vi "LSMcontroller_v58.vi"() -> ()   [LabVIEW 2015] (continued)
                                n1730 = Divide(x=1.0 ("Digital DC (%)"), y=w4415) -> (x/y=w4417:dbl)
                                n1731 = Multiply(x=100.0, y=w4417) -> (x*y=w4414:dbl)
                                n1732 = Bundle By Name(cluster=w4431, "Digital DC (%)"=w4414, "Digital phase"=w4426, "Digital Freq (Hz)"=w4422, "Sampling frequency (Hz)"=w4419, "Digital time offset (s)"=w4426, "padding value"=0.0, "matlab wave file"=path "LT", "DOtab"=0.0) -> (w4429:T20)
                                n1733 = Build Array(w4429) -> (w4428:T19)
                                n1734 = call "waveformparamsv2.vi"("command"="add DO", "add DO"=w4428) -> ()  [unwired: 3 in, 3 out]
                                }
                                frame 2 {
                                n1735 = call "waveformparamsv2.vi"("command"="get") -> ("Params out"=w4441:T16)  [unwired: 4 in, 2 out]
                                n1736 = in-place {
                                in-place-border: w4439 -> [w4445]
                                in-place-border: [w4444] -> w4438
                                n1737 = in-place-cluster #30(w4441) -> ("DO parameters"=w4447:T19)
                                n1738 = Delete From Array(array=w4447, length=1, index=w4445) -> (deleted portion=w4444:T19, array with subset deleted=w4446:T19)
                                n1739 = in-place-cluster #30("DO parameters"=w4446) -> (w4440:T16)
                                }
                                n1740 = call "waveformparamsv2.vi"("command"="set", "Params in"=w4440) -> ()  [unwired: 3 in, 3 out]
                                }
                                frame 3, Default {
                                }
                                frame 0 {
                                n1741 = local read "Measurement"() -> (w4453:T5)
                                n1742 = To Unsigned Long Integer(number=w4453) -> (unsigned 32bit integer=w4452:u32)
                                n1743 = case shown="5..7" w4452 {
                                tunnel: w4451 -> [_ w4455]
                                tunnel: [_ w4454] -> w4450
                                frame 0..4, Default {
                                }
                                frame 5..7 {
                                n1744 = stacked-sequence {
                                tunnel: w4455 -> [w4457 w4466]
                                tunnel: [w4456 _] -> w4454
                                frame #0 {
                                n1745 = call "waveformparamsv2.vi"("command"="get") -> ("Params out"=w4459:T16)  [unwired: 4 in, 2 out]
                                n1746 = Unbundle By Name(w4459) -> ("DO parameters"=w4460:T19)
                                n1747 = Index Array(array=w4460, index=w4457) -> (element=w4456:T20)
                                }
                                frame #1 {
                                w4474 = 0.0 ("padding value")
                                n1748 = call "2pparameters.vi"("command"="get") -> ("params out"=w4472:T12)  [unwired: 1 in]
                                n1749 = Unbundle By Name(w4472) -> ("srate"=w4470:sgl, "Pel"=w4471:sgl)
                                n1750 = To Double Precision Float(number=w4470) -> (double precision float=w4468:dbl)
                                n1751 = To Double Precision Float(number=w4470) -> (double precision float=w4469:dbl)
                                n1752 = To Double Precision Float(number=w4471) -> (double precision float=w4464:dbl)
                                n1753 = Divide(x=1.0 ("Digital DC (%)"), y=w4464) -> (x/y=w4463:dbl)
                                n1754 = Multiply(x=100.0, y=w4463) -> (x*y=w4462:dbl)
                                n1755 = Divide(x=w4469, y=w4464) -> (x/y=w4467:dbl)
                                n1756 = call "replace DO wf param.vi"("Digital Freq (Hz)"=w4467, "Digital DC (%)"=w4462, "Digital phase"=w4474, "Sampling frequency (Hz)"=w4468, "Digital time offset (s)"=w4474, "index of DO wave"=w4466, "padding value"=w4474, "matlab wave file"=path "LT" ("matlab wave number")) -> ()  [unwired: 3 in]
                                }
                                }
                                }
                                }
                                n1757 = Build Array(w4450) -> (w4449:T19)
                                }
                                }
                                }
                                frame #9 {
                                n1758 = Build Array(w4479, w4478) -> (w4481:bool[])
                                n1759 = Boolean Array To Number(Boolean array=w4481) -> (number=w4480:u32)
                                n1760 = case shown="0" w4480 {
                                tunnel: w4477 -> [_ w4533 _ w4537]
                                tunnel: [_ w4528 _ w4534] -> w4476
                                frame 1 {
                                n1761 = call "2pparameters.vi"("command"="get") -> ("params out"=w4488:T12)  [unwired: 1 in]
                                n1762 = Unbundle By Name(w4488) -> ("wavdet"=w4489:bool, "Pel"=w4491:sgl, "refwfsize"=w4492:dbl, "Pel"=w4490:sgl)
                                n1763 = call "waveformsDObuffer.vi"("command"="get") -> ("DO wf out"=w4484:digitalwaveform[])  [unwired: 1 in]
                                n1764 = case shown="True" w4489 {
                                tunnel: [w4496 w4509] -> w4486
                                tunnel: w4490 -> [w4505 w4524]
                                tunnel: w4491 -> [w4495 w4515]
                                tunnel: w4492 -> [_ w4521]
                                frame False {
                                w4499 = u16 0 items=["unsigned binary", "offset binary", "2's complement"] ("data format (offset binary)")
                                n1765 = Initialize Array(sgl 0.0, w4495) -> (w4502:sgl[])
                                n1766 = Replace Array Subset(array=w4502, new element=sgl 1.0, index=0) -> (w4500:sgl[])
                                n1767 = Reciprocal(x=w4505) -> (1/x=w4506:sgl)
                                n1768 = Bundle By Name("Y"=w4500, "dt"=w4506) -> (w4497:waveform(sgl))  [unwired: 1 in]
                                n1769 = call-poly <vilib>:"Analog to Digital.vi"("data format (offset binary)"=w4499, "compress digital (T)"=TRUE, "full-scale range (pk-pk)"=1.0, "resolution (16 bit)"=1, "analog waveform"=w4497) -> ("digital waveform"=w4496:digitalwaveform)  [unwired: 3 in, 3 out]
                                }
                                frame True {
                                w4512 = u16 0 items=["unsigned binary", "offset binary", "2's complement"] ("data format (offset binary)")
                                n1770 = To Double Precision Float(number=w4515) -> (double precision float=w4522:dbl)
                                n1771 = Initialize Array(sgl 0.0, w4515) -> (w4517:sgl[])
                                n1772 = Divide(x=w4521, y=w4522) -> (x/y=w4519:dbl)
                                n1773 = Round Toward +Infinity(x=w4519) -> (ceil(x): smallest int >= x=w4520:dbl)
                                n1774 = Replace Array Subset(array=w4517, new element=sgl 1.0, index=0) -> (w4514:sgl[])
                                n1775 = for {
                                N: w4520 -> [_]
                                tunnel: w4514 -> [w4526]
                                tunnel: [w4526] -> w4523 mode=concatenating
                                }
                                n1776 = Reciprocal(x=w4524) -> (1/x=w4525:sgl)
                                n1777 = Bundle By Name("Y"=w4523, "dt"=w4525) -> (w4510:waveform(sgl))  [unwired: 1 in]
                                n1778 = call-poly <vilib>:"Analog to Digital.vi"("data format (offset binary)"=w4512, "compress digital (T)"=TRUE, "full-scale range (pk-pk)"=1.0, "resolution (16 bit)"=1, "analog waveform"=w4510) -> ("digital waveform"=w4509:digitalwaveform)  [unwired: 3 in, 3 out]
                                }
                                }
                                n1779 = Build Array (concatenate)(w4484, w4486) -> (w4482:digitalwaveform[])
                                n1780 = call "waveformsDObuffer.vi"("DO wf in"=w4482, "command"="set") -> ()  [unwired: 1 out]
                                }
                                frame 2 {
                                n1781 = call "waveformsDObuffer.vi"("command"="get") -> ("DO wf out"=w4530:digitalwaveform[])  [unwired: 1 in]
                                n1782 = Delete From Array(array=w4530, length=1, index=w4533) -> (deleted portion=w4528:digitalwaveform[], array with subset deleted=w4527:digitalwaveform[])
                                n1783 = call "waveformsDObuffer.vi"("DO wf in"=w4527, "command"="set") -> ()  [unwired: 1 out]
                                }
                                frame 3, Default {
                                }
                                frame 0 {
                                n1784 = local read "Measurement"() -> (w4536:T5)
                                n1785 = To Unsigned Long Integer(number=w4536) -> (unsigned 32bit integer=w4535:u32)
                                n1786 = case shown="5..7" w4535 {
                                tunnel: w4537 -> [_ w4540]
                                tunnel: [_ w4539] -> w4534
                                frame 0..4, Default {
                                }
                                frame 5..7 {
                                n1787 = call "2pparameters.vi"("command"="get") -> ("params out"=w4547:T12)  [unwired: 1 in]
                                n1788 = Unbundle By Name(w4547) -> ("wavdet"=w4548:bool, "Pel"=w4550:sgl, "refwfsize"=w4551:dbl, "srateAODO"=w4549:sgl)
                                n1789 = call "waveformsDObuffer.vi"("command"="get") -> ("DO wf out"=w4541:digitalwaveform[])  [unwired: 1 in]
                                n1790 = Index Array(array=w4541, index=w4540) -> (element=w4542:digitalwaveform)
                                n1791 = case shown="True" w4548 {
                                tunnel: [w4555 w4568] -> w4545
                                tunnel: w4549 -> [w4564 w4583]
                                tunnel: w4550 -> [w4554 w4574]
                                tunnel: w4551 -> [_ w4580]
                                frame False {
                                w4558 = u16 0 items=["unsigned binary", "offset binary", "2's complement"] ("data format (offset binary)")
                                n1792 = Initialize Array(sgl 0.0, w4554) -> (w4561:sgl[])
                                n1793 = Replace Array Subset(array=w4561, new element=sgl 1.0, index=0) -> (w4559:sgl[])
                                n1794 = Reciprocal(x=w4564) -> (1/x=w4565:sgl)
                                n1795 = Bundle By Name("Y"=w4559, "dt"=w4565) -> (w4556:waveform(sgl))  [unwired: 1 in]
                                n1796 = call-poly <vilib>:"Analog to Digital.vi"("data format (offset binary)"=w4558, "compress digital (T)"=TRUE, "full-scale range (pk-pk)"=1.0, "resolution (16 bit)"=1, "analog waveform"=w4556) -> ("digital waveform"=w4555:digitalwaveform)  [unwired: 3 in, 3 out]
                                }
                                frame True {
                                w4571 = u16 0 items=["unsigned binary", "offset binary", "2's complement"] ("data format (offset binary)")
                                n1797 = To Double Precision Float(number=w4574) -> (double precision float=w4581:dbl)
                                n1798 = Initialize Array(sgl 0.0, w4574) -> (w4576:sgl[])
                                n1799 = Divide(x=w4580, y=w4581) -> (x/y=w4578:dbl)
                                n1800 = Round Toward +Infinity(x=w4578) -> (ceil(x): smallest int >= x=w4579:dbl)
                                n1801 = Replace Array Subset(array=w4576, new element=sgl 1.0, index=0) -> (w4573:sgl[])
                                n1802 = for {
                                N: w4579 -> [_]
                                tunnel: w4573 -> [w4585]
                                tunnel: [w4585] -> w4582 mode=concatenating
                                }
                                n1803 = Reciprocal(x=w4583) -> (1/x=w4584:sgl)
                                n1804 = Bundle By Name("Y"=w4582, "dt"=w4584) -> (w4569:waveform(sgl))  [unwired: 1 in]
                                n1805 = call-poly <vilib>:"Analog to Digital.vi"("data format (offset binary)"=w4571, "compress digital (T)"=TRUE, "full-scale range (pk-pk)"=1.0, "resolution (16 bit)"=1, "analog waveform"=w4569) -> ("digital waveform"=w4568:digitalwaveform)  [unwired: 3 in, 3 out]
                                }
                                }
                                n1806 = Build Array(w4542) -> (w4539:digitalwaveform[])
                                n1807 = Replace Array Subset(array=w4541, new element=w4545, index=w4540) -> (w4538:digitalwaveform[])
                                n1808 = call "waveformsDObuffer.vi"("DO wf in"=w4538, "command"="set") -> ()  [unwired: 1 out]
                                }
                                }
                                }
                                }
                                }
                                frame #10 {
                                n1809 = local read "Meastab"() -> (w4599:enum32{"X-Y Image", "Linescan", "Timetrace"})
                                n1810 = property on="refwf" class="Ring (strict)"() -> ("RingText.Text"=w4596:string)  [unwired: 2 in, 2 out]
                                n1811 = case shown="\"Timetrace\"" w4599 {
                                tunnel: [w4601 w4602] -> w4600
                                frame "X-Y Image", Default {
                                n1812 = local read "Sampling rate"() -> (w4601:dbl)
                                }
                                frame "Timetrace" {
                                n1813 = local read "srateAODOtt"() -> (w4602:dbl)
                                }
                                }
                                n1814 = call "waveformsAObuffer.vi"("command"="get") -> ("AO wf out"=w4589:waveform(dbl)[])  [unwired: 1 in]
                                n1815 = local read "wavdet"() -> (w4597:bool)
                                n1816 = call "waveformsDObuffer.vi"("command"="get") -> ("DO wf out"=w4593:digitalwaveform[])  [unwired: 1 in]
                                n1817 = call "correctwaveformsizetemp.vi"("new sampling frequency (Hz)"=w4600, "start"=TRUE, "reference waveforms to"=w4596, "Analog waveforms in"=w4589, "stop"=FALSE, "Digital waveforms in"=w4593) -> ("analog wf out"=w4595:waveform(dbl)[], "Digital wf out"=w4588:digitalwaveform[], "measpoints"=w4598:i32)
                                n1818 = call "waveformsDObuffer.vi"("DO wf in"=w4588, "command"="set") -> ()  [unwired: 1 out]
                                n1819 = call "waveformsAObuffer.vi"("AO wf in"=w4595, "command"="set") -> ()  [unwired: 1 out]
                                n1820 = case shown="True" w4597 {
                                tunnel: w4598 -> [_ w4605]
                                tunnel: w4588 -> [_ w4603]
                                frame False {
                                }
                                frame True {
                                n1821 = local write "# of frames"(w4605) -> ()
                                n1822 = call "GetNumCamFramesv2.vi"("Digital Waveform Graph"=w4603) -> ("Numeric"=w4604:i32)  [unwired: 10 in]
                                n1823 = local write "Total Camera Frames"(w4604) -> ()
                                }
                                }
                                }
                                }
                              }
                              frame #7 {
                                # "Disabled for conversion to 64 bit"
                                n1824 = disable-structure shown="Disabled" {
                                frame Disabled {
                                n1825 = local read "Measurement"() -> (w4607:T5)
                                n1826 = case shown="\"Lifetime (scan)\"" w4607 {
                                frame "X-Y-t movie", Default {
                                }
                                frame "Lifetime (scan)" {
                                # "total acquisition time"
                                n1827 = call "2pparameters.vi"("command"="get") -> ("params out"=w4615:T12)  [unwired: 1 in]
                                n1828 = Unbundle By Name(w4615) -> ("measpoints"=w4609:i32, "srateAODO"=w4630:sgl)
                                n1829 = Divide(x=w4609, y=w4630) -> (x/y=w4608:sgl)
                                n1830 = local read "min phot"() -> (w4625:u32)
                                n1831 = local read "expected c/s"() -> (w4626:dbl)
                                n1832 = Multiply(x=w4608, y=1000.0) -> (x*y=w4618:dbl)
                                n1833 = local read "Ch1 ZeroX"() -> (w4623:i32)
                                n1834 = local read "truncate"() -> (w4624:u32)
                                n1835 = To Long Integer(number=w4618) -> (32bit integer=w4627:i32)
                                n1836 = To Long Integer(number=w4626) -> (32bit integer=w4628:i32)
                                n1837 = local read "Number of Bins"() -> (w4619:u32)
                                n1838 = local read "Ch1 Level"() -> (w4621:i32)
                                n1839 = local read "Ch0 ZeroX"() -> (w4622:i32)
                                n1840 = local write "Acquisition time"(w4627) -> ()
                                n1841 = local read "Ch0 Level"() -> (w4620:i32)
                                n1842 = call "lifetimeparameters.vi"("command"="get") -> ("Params out"=w4613:T21)  [unwired: 1 in]
                                n1843 = Add(x=100, y=w4627) -> (x+y=w4617:i32)
                                n1844 = Bundle By Name(cluster=w4613, "acq time"=w4617, "acq rate"=w4628, "# bins"=w4619, "Ch0 Level"=w4620, "Ch1 Level"=w4621, "Ch0 ZeroX"=w4622, "Ch1 ZeroX"=w4623, "min photons"=w4625, "truncate"=w4624) -> (w4612:T21)
                                n1845 = local write "Acquisition rate"(w4628) -> ()
                                n1846 = call "lifetimeparameters.vi"("Params in"=w4612, "command"="set") -> ()  [unwired: 1 out]
                                }
                                }
                                }
                                frame Enabled {
                                }
                                }
                                n1847 = local write "64bit disabled"(TRUE ("64bit disabled")) -> ()
                              }
                              frame #8 {
                                n1848 = call "2pparameters.vi"("command"="get") -> ("params out"=w4641:T12)  [unwired: 1 in]
                                n1849 = Unbundle By Name(w4641) -> ("refreshbuffer"=w4639:i32, "srate"=w4640:sgl)
                                n1850 = local read "wavdet"() -> (w4631:bool)
                                n1851 = To Double Precision Float(number=w4640) -> (double precision float=w4643:dbl)
                                n1852 = To Double Precision Float(number=w4639) -> (double precision float=w4634:dbl)
                                n1853 = case shown="False" w4631 {
                                tunnel: [w4648 w4649] -> w4633
                                frame False {
                                w4648 = 10123 items=["Finite Samples"=10178, "Continuous Samples"=10123, "Hardware Timed Single Point"=12522] ("sample mode")
                                }
                                frame True {
                                w4649 = 10123 items=["Finite Samples"=10178, "Continuous Samples"=10123, "Hardware Timed Single Point"=12522] ("sample mode")
                                }
                                }
                                n1854 = Divide(x=w4634, y=w4643) -> (x/y=w4647:dbl)
                                n1855 = Multiply(x=w4647, y=2.0) -> (x*y=w4644:dbl)
                                n1856 = Max & Min(x=w4644, y=10.0) -> (max(x,y)=w4635:dbl)  [unwired: 1 out]
                                n1857 = call "2pparameters.vi"("command"="get") -> ("params out"=w4638:T12)  [unwired: 1 in]
                                n1858 = Bundle By Name(cluster=w4638, "timeout"=w4635, "sample mode"=w4633) -> (w4636:T12)
                                n1859 = call "2pparameters.vi"("Params in"=w4636, "command"="set") -> ()  [unwired: 1 out]
                              }
                            }
                          }
                          frame #1 {
                            # "Disabled for conversion to 64 bit"
                            n1860 = call "prepAO_img.vi"() -> ("Terminal Name with Device Prefix"=w4651:tag)
                            n1861 = call "prepDO_img.vi"() -> ()  [unwired: 2 in]
                            n1862 = call "prepAI_img.vi"("triggersource"=w4651) -> ()  [unwired: 2 in]
                            n1863 = call "prepCI_img.vi"("ArmStart.DigEdge.Src"=w4651) -> ()  [unwired: 1 in]
                            n1864 = disable-structure shown="Disabled" {
                              frame Disabled {
                                n1865 = local read "Measurement"() -> (w4652:T5)
                                n1866 = case shown="\"Lifetime (contour)\"" w4652 {
                                frame "X-Y-t movie", Default {
                                }
                                frame "Lifetime (contour)" {
                                n1867 = stacked-sequence {
                                frame #0 {
                                n1868 = call "PH-temp.vi"("String"="clear" ("command")) -> ()  [unwired: 2 in, 2 out]
                                n1869 = call "PH-temp-raw.vi"("command"="empty") -> ()  [unwired: 1 in, 1 out]
                                }
                                frame #1 {
                                n1870 = call "calib.vi"() -> ()  [unwired: 1 in]
                                }
                                frame #2 {
                                n1871 = call "setup.vi"() -> ()  [unwired: 1 in]
                                }
                                }
                                }
                                }
                              }
                              frame Enabled {
                              }
                            }
                            n1872 = local write "64bit disabled"(TRUE ("64bit disabled")) -> ()
                          }
                          frame #2 {
                            n1873 = local read "save\ndata"() -> (w4655:bool)
                            n1874 = case shown="True" w4655 {
                              tunnel: w4656 -> [_ w4660]
                              frame False {
                              }
                              frame True {
                                n1875 = local read "filename prefix"() -> (w4658:string)
                                n1876 = local read "data dir"() -> (w4659:path)
                                n1877 = call "preparebinaryfiles.vi"("filename prefix"=w4658, "data dir"=w4659, "timestamp"=w4660) -> ("full-filename"=w4657:string)  [unwired: 1 in]
                                n1878 = local write "full-filename"(w4657) -> ()
                              }
                            }
                            n1879 = call "preptempbuffers_tt.vi"() -> ()  [unwired: 12 in]
                          }
                          frame #3 {
                            n1880 = local read "wavdet"() -> (w4661:bool)
                            n1881 = case shown="False" w4661 {
                              frame False {
                                n1882 = disable-structure shown="Disabled" {
                                frame Disabled {
                                n1883 = call "2pparameters.vi"("command"="get") -> ("params out"=w4663:T12)  [unwired: 1 in]
                                n1884 = Unbundle By Name(w4663) -> ("autoshutter"=w4664:bool)
                                n1885 = case shown="True" w4664 {
                                frame False {
                                }
                                frame True {
                                n1886 = call "shuttercontrol.vi"("command"="open") -> ()  [unwired: 1 in, 1 out]
                                }
                                }
                                }
                                frame Enabled {
                                }
                                }
                              }
                              frame True {
                              }
                            }
                          }
                          frame #4 {
                            n1887 = flat-sequence {
                              frame #0 {
                                # "Disabled for conversion to 64 bit"
                                n1888 = disable-structure shown="Disabled" {
                                frame Disabled {
                                n1889 = local read "Measurement"() -> (w4667:T5)
                                n1890 = case shown="\"Lifetime (contour)\"" w4667 {
                                frame "X-Y-t movie", Default {
                                }
                                frame "Lifetime (contour)" {
                                n1891 = call "runLT_img.vi"() -> ()  [unwired: 1 in]
                                }
                                }
                                }
                                frame Enabled {
                                }
                                }
                                n1892 = local write "64bit disabled"(TRUE ("64bit disabled")) -> ()
                              }
                              frame #1 {
                                n1893 = call "runAI_img.vi"() -> ()  [unwired: 12 in]
                                n1894 = call "runCI.vi"() -> ()  [unwired: 12 in]
                                n1895 = call "runDO_img.vi"() -> ()  [unwired: 12 in]
                              }
                              frame #2 {
                                n1896 = call "runAO_img.vi"() -> ()  [unwired: 12 in]
                              }
                            }
                          }
                          frame #5 {
                            # "Disabled for conversion to 64 bit"
                            n1897 = disable-structure shown="Disabled" {
                              disable-tunnel: w4669 -> [w4670 _]
                              frame Disabled {
                                w4673 = u16 0 items=["Stream to disk", "Post process", "real time process"] ("Ring")
                                n1898 = local read "T3R Data processing"() -> (w4672:u16)
                                n1899 = Equal?(x=w4672, y=w4673) -> (x = y?=w4671:bool)
                                n1900 = local read "save\ndata"() -> (w4675:bool)
                                n1901 = local read "Measurement"() -> (w4676:T5)
                                n1902 = And(x=w4675, y=w4671) -> (x .and. y?=w4674:bool)
                                n1903 = case shown="\"Lifetime (contour)\"" w4676 {
                                tunnel: w4670 -> [_ w4680]
                                tunnel: w4674 -> [_ w4678]
                                frame "X-Y-t movie", Default {
                                }
                                frame "Lifetime (contour)" {
                                n1904 = case shown="True" w4678 {
                                selector: w4678 -> [w4681 w4686]
                                tunnel: w4680 -> [_ w4684]
                                tunnel: [path "" ("appended path") w4687] -> w4679
                                tunnel: [w4681 w4686] -> w4677
                                frame False {
                                }
                                frame True {
                                n1905 = local read "filename prefix"() -> (w4685:string)
                                n1906 = local read "data dir"() -> (w4688:path)
                                n1907 = call "generatedatafilename.vi"("timestamp"=w4684, "filename prefix in"=w4685) -> ("full-filename"=w4683:string)
                                n1908 = Concatenate Strings(w4683, ".lvpt3contour" ("string")) -> (w4690:string)
                                n1909 = Build Path(base path=w4688, name or relative path=w4690) -> (appended path=w4687:path)
                                }
                                }
                                n1910 = call "collectLT_res_v1.vi"("stream?"=w4677, "data file"=w4679) -> ()  [unwired: 2 out]
                                }
                                }
                              }
                              frame Enabled {
                              }
                            }
                            n1911 = while {
                              i -> [w4693]
                              stop <- w4691 stop-if-true
                              n1912 = local read "Stop"() -> (w4701:bool)
                              n1913 = local read "Exit"() -> (w4700:bool)
                              n1914 = Increment(x=w4693) -> (x+1=w4692:i32)
                              n1915 = local write "points recorded"(w4692) -> ()
                              n1916 = Or(x=w4701, y=w4700) -> (x .or. y?=w4699:bool)
                              n1917 = case shown="False" w4699 {
                                frame False {
                                n1918 = stacked-sequence {
                                frame #0 {
                                n1919 = call "collectAI_tt_V2.vi"() -> ()  [unwired: 4 in]
                                n1920 = call "collectCI_tt.vi"() -> ("size(s)"=w4708:i32)  [unwired: 3 in]
                                n1921 = local write "scol"(w4708) -> ()
                                }
                                frame #1 {
                                n1922 = local read "Live"() -> (w4709:bool)
                                n1923 = case shown="True" w4709 {
                                frame False {
                                }
                                frame True {
                                n1924 = local read "graph1list"() -> (w4716:u16)
                                n1925 = local read "graph2list"() -> (w4715:u16)
                                n1926 = To Unsigned Word Integer(number=w4716) -> (unsigned 16bit integer=w4714:u16)
                                n1927 = To Unsigned Word Integer(number=w4715) -> (unsigned 16bit integer=w4713:u16)
                                n1928 = call "dattotrace.vi"("graph2list"=w4713, "Current Average"=sgl 1.0, "graph1list"=w4714) -> ("trace2array out"=w4711:sgl[], "trace1array out"=w4722:sgl[])
                                n1929 = local read "bin"() -> (w4723:dbl)
                                n1930 = script code="data=reshape(datain,[bin length(datain)./bin]);\ndataout=mean(data,1);\ndata2=reshape(datain2,[bin length(datain2)./bin]);\ndataout2=mean(data2,1);"("bin"=w4723, "datain"=w4722, "datain2"=w4711) -> ("dataout"=w4721:dbl[], "dataout2"=w4710:dbl[])  [unwired: 1 in, 1 out]
                                n1931 = Array Size(array=w4710) -> (size(s)=w4724:i32)
                                n1932 = Divide(x=w4724, y=2) -> (x/y=w4726:dbl)
                                n1933 = Round To Nearest(number=w4726) -> (nearest integer value=w4728:dbl)
                                n1934 = Array Size(array=w4721) -> (size(s)=w4733:i32)
                                n1935 = Delete From Array(array=w4710, length=w4728, index=0) -> (deleted portion=w4719:dbl[], array with subset deleted=w4720:dbl[])
                                n1936 = Divide(x=w4733, y=2) -> (x/y=w4731:dbl)
                                n1937 = Round To Nearest(number=w4731) -> (nearest integer value=w4729:dbl)
                                n1938 = Delete From Array(array=w4721, length=w4729, index=0) -> (deleted portion=w4718:dbl[], array with subset deleted=w4717:dbl[])
                                n1939 = local write "graph2"(w4717) -> ()
                                n1940 = local write "graph1"(w4718) -> ()
                                n1941 = local write "graph3"(w4719) -> ()
                                n1942 = local write "graph4"(w4720) -> ()
                                }
                                }
                                }
                                frame #2 {
                                n1943 = local read "save\ndata"() -> (w4734:bool)
                                n1944 = case shown="True" w4734 {
                                frame False {
                                }
                                frame True {
                                n1945 = call "savebinaryfiles.vi"() -> ()  [unwired: 1 in]
                                }
                                }
                                }
                                }
                                }
                                frame True {
                                }
                              }
                              n1946 = local read "continuous"() -> (w4696:bool)
                              n1947 = case shown="False" w4696 {
                                tunnel: w4692 -> [w4706 _]
                                tunnel: [w4705 FALSE] -> w4694
                                frame False {
                                n1948 = call "2pparameters.vi"("command"="get") -> ("params out"=w4703:T12)  [unwired: 1 in]
                                n1949 = Unbundle By Name(w4703) -> ("tt_cycles"=w4702:i32)
                                n1950 = Greater Or Equal?(x=w4706, y=w4702) -> (x >= y?=w4705:bool)
                                }
                                frame True {
                                }
                              }
                              n1951 = local read "Stop"() -> (w4698:bool)
                              n1952 = local read "Exit"() -> (w4697:bool)
                              n1953 = Or(x=w4698, y=w4697) -> (x .or. y?=w4695:bool)
                              n1954 = Or(x=w4695, y=w4694) -> (x .or. y?=w4691:bool)
                            }
                            n1955 = local write "64bit disabled"(TRUE ("64bit disabled")) -> ()
                          }
                          frame #6 {
                            # "Disabled for conversion to 64 bit"
                            n1956 = local read "Measurement"() -> (w4737:T5)
                            n1957 = disable-structure shown="Disabled" {
                              disable-tunnel: w4737 -> [w4739 _]
                              disable-tunnel: w4736 -> [w4738 _]
                              frame Disabled {
                                n1958 = case shown="\"Lifetime (contour)\"" w4739 {
                                tunnel: w4738 -> [_ w4740]
                                frame "X-Y-t movie", Default {
                                }
                                frame "Lifetime (contour)" {
                                n1959 = stacked-sequence {
                                tunnel: w4740 -> [_ w4741]
                                frame #0 {
                                n1960 = flat-sequence {
                                frame #0 {
                                n1961 = call "stoperaseLT_img.vi"() -> ()  [unwired: 1 in]
                                }
                                }
                                }
                                frame #1 {
                                w4744 = u16 0 items=["Stream to disk", "Post process", "real time process"] ("Ring")
                                n1962 = local read "T3R Data processing"() -> (w4743:u16)
                                n1963 = local read "save\ndata"() -> (w4746:bool)
                                n1964 = Equal?(x=w4743, y=w4744) -> (x = y?=w4742:bool)
                                n1965 = Not(x=w4742) -> (.not. x?=w4747:bool)
                                n1966 = And(x=w4746, y=w4747) -> (x .and. y?=w4745:bool)
                                n1967 = case shown="True" w4745 {
                                tunnel: w4741 -> [_ w4748]
                                frame False {
                                }
                                frame True {
                                n1968 = local read "filename prefix"() -> (w4749:string)
                                n1969 = local read "data dir"() -> (w4765:path)
                                n1970 = call "2pparameters.vi"("command"="get") -> ("params out"=w4760:T12)  [unwired: 1 in]
                                n1971 = call "generatedatafilename.vi"("timestamp"=w4748, "filename prefix in"=w4749) -> ("full-filename"=w4750:string)
                                n1972 = Unbundle By Name(w4760) -> ("srate"=w4758:sgl, "Pel"=w4757:sgl, "measpoints"=w4755:i32)
                                n1973 = Concatenate Strings(w4750, ".lvpt3contour" ("string")) -> (w4763:string)
                                n1974 = Build Path(base path=w4765, name or relative path=w4763) -> (appended path=w4762:path)
                                n1975 = To Unsigned Long Integer(number=w4758) -> (unsigned 32bit integer=w4759:u32)
                                n1976 = To Unsigned Long Integer(number=w4757) -> (unsigned 32bit integer=w4756:u32)
                                n1977 = To Unsigned Long Integer(number=w4755) -> (unsigned 32bit integer=w4754:u32)
                                n1978 = call "PH-temp-raw.vi"("command"="get") -> ("array out"=w4753:u32[])  [unwired: 1 in]
                                n1979 = Build Array (concatenate)(w4759, w4756, w4754, w4753) -> (w4752:u32[])
                                n1980 = Open/Create/Replace File(file path (use dialog)=w4762, operation (0:open)=T9."replace or create") -> (refnum out=w4769:refnum<file>, error out=w4768:errorcluster)  [unwired: 4 in, 1 out]
                                n1981 = Write to Binary File(file (use dialog)=w4769, data=w4752, error in=w4768, 5:FALSE ("prepend array or string size? (T)")) -> (refnum out=w4766:refnum<file>, error out=w4767:errorcluster)  [unwired: 2 in, 1 out]
                                n1982 = Close File(refnum=w4766, error in=w4767) -> ()  [unwired: 2 out]
                                }
                                }
                                }
                                }
                                }
                                }
                              }
                              frame Enabled {
                              }
                            }
                            n1983 = local write "64bit disabled"(TRUE ("64bit disabled")) -> ()
                          }
                          frame #7 {
                            n1984 = call "reset AO_DO_v3.vi"() -> ()  [unwired: 12 in]
                          }
                          frame #8 {
                            n1985 = stacked-sequence {
                              tunnel: w4785 -> [w4788 _ _ _ _ _]
                              tunnel: w4782 -> [w4787 _ _ _ _ _]
                              tunnel: w4783 -> [w4786 _ _ _ _ _]
                              tunnel: w4784 -> [_ w4837 _ _ _ _]
                              tunnel: w4780 -> [_ w4836 w4891 w4988 _ _]
                              tunnel: w4781 -> [_ w4835 w4890 w4987 _ _]
                              tunnel: w4779 -> [_ _ _ w4986 _ _]
                              tunnel: w4778 -> [_ _ _ w4985 _ _]
                              tunnel: w4777 -> [_ _ w4888 _ _ _]
                              tunnel: w4776 -> [_ _ w4887 _ _ _]
                              tunnel: w4775 -> [_ _ w4885 _ _ _]
                              tunnel: w4774 -> [_ _ w4884 _ _ _]
                              tunnel: w4773 -> [_ _ _ w4983 _ _]
                              tunnel: w4772 -> [_ _ _ w4982 _ _]
                              frame #0 {
                                n1986 = case shown="False" w4788 {
                                tunnel: w4787 -> [_ w4810]
                                tunnel: w4786 -> [_ w4809]
                                frame True {
                                n1987 = stacked-sequence {
                                seq-local: [w4789 _ _] -> [_ w4801 w4806]
                                frame #0 {
                                n1988 = call "configuration.vi"("command"="get") -> ("config out"=w4795:T13)  [unwired: 2 in, 1 out]
                                n1989 = Unbundle By Name(w4795) -> ("Voltage to Xgalvo"=w4792:i32)
                                n1990 = call "2pparameters.vi"("command"="get") -> ("params out"=w4793:T12)  [unwired: 1 in]
                                n1991 = in-place {
                                in-place-border: w4792 -> [w4800]
                                in-place-border: [w4797] -> w4789
                                n1992 = in-place-cluster #31(w4793) -> ("aAO"=w4799:u32[])
                                n1993 = call "remove channel from active arrayv2.vi"("line array in"=w4799, "line to remove"=w4800) -> ("line array out"=w4798:u32[], "index"=w4797:i32)  [unwired: 1 out]
                                n1994 = in-place-cluster #31("aAO"=w4798) -> (w4790:T12)
                                }
                                n1995 = call "2pparameters.vi"("Params in"=w4790, "command"="set") -> ()  [unwired: 1 out]
                                }
                                frame #1 {
                                n1996 = call "waveformparamsv2.vi"("command"="rem AO", "index"=w4801) -> ()  [unwired: 3 in, 3 out]
                                }
                                frame #2 {
                                n1997 = call "waveformsAObuffer.vi"("command"="get") -> ("AO wf out"=w4807:waveform(dbl)[])  [unwired: 1 in]
                                n1998 = Delete From Array(array=w4807, length=1, index=w4806) -> (array with subset deleted=w4803:waveform(dbl)[])  [unwired: 1 out]
                                n1999 = call "waveformsAObuffer.vi"("AO wf in"=w4803, "command"="set") -> ()  [unwired: 1 out]
                                }
                                }
                                }
                                frame False {
                                n2000 = stacked-sequence {
                                seq-local: [w4811 _ _] -> [_ w4819 w4830]
                                tunnel: w4810 -> [_ w4818 _]
                                tunnel: w4809 -> [_ _ w4829]
                                frame #0 {
                                n2001 = call "configuration.vi"("command"="get") -> ("config out"=w4816:T13)  [unwired: 2 in, 1 out]
                                n2002 = Unbundle By Name(w4816) -> ("Voltage to Xgalvo"=w4812:i32)
                                n2003 = call "2pparameters.vi"("command"="get") -> ("params out"=w4815:T12)  [unwired: 1 in]
                                n2004 = Unbundle By Name(w4815) -> ("aAO"=w4813:u32[])
                                n2005 = Search 1D Array(1D array=w4813, element=w4812) -> (index of element=w4811:i32)  [unwired: 1 in]
                                }
                                frame #1 {
                                n2006 = call "waveformparamsv2.vi"("command"="get") -> ("Params out"=w4822:T16)  [unwired: 4 in, 2 out]
                                n2007 = in-place {
                                in-place-border: w4819 -> [w4826]
                                in-place-border: w4818 -> [w4825]
                                n2008 = in-place-cluster #32(w4822) -> ("AO parameters"=w4827:T17)
                                n2009 = in-place {
                                in-place-border: w4825 -> [w4828]
                                n2010 = in-place-array #33(w4827, w4826) -> ()  [unwired: 1 out]
                                n2011 = in-place-array #33(w4828) -> (w4824:T17)  [unwired: 1 out]
                                }
                                n2012 = in-place-cluster #32("AO parameters"=w4824) -> (w4820:T16)
                                }
                                n2013 = call "waveformparamsv2.vi"("command"="set", "Params in"=w4820) -> ()  [unwired: 3 in, 3 out]
                                }
                                frame #2 {
                                n2014 = call "waveformsAObuffer.vi"("command"="get") -> ("AO wf out"=w4833:waveform(dbl)[])  [unwired: 1 in]
                                n2015 = Replace Array Subset(array=w4833, new element=w4829, index=w4830) -> (w4831:waveform(dbl)[])
                                n2016 = call "waveformsAObuffer.vi"("AO wf in"=w4831, "command"="set") -> ()  [unwired: 1 out]
                                }
                                }
                                }
                                }
                              }
                              frame #1 {
                                n2017 = case shown="False" w4837 {
                                tunnel: w4836 -> [_ w4859]
                                tunnel: w4835 -> [_ w4858]
                                frame True {
                                n2018 = stacked-sequence {
                                seq-local: [w4838 _ _] -> [_ w4850 w4855]
                                frame #0 {
                                n2019 = call "configuration.vi"("command"="get") -> ("config out"=w4844:T13)  [unwired: 2 in, 1 out]
                                n2020 = Unbundle By Name(w4844) -> ("Voltage to Ygalvo"=w4841:i32)
                                n2021 = call "2pparameters.vi"("command"="get") -> ("params out"=w4842:T12)  [unwired: 1 in]
                                n2022 = in-place {
                                in-place-border: w4841 -> [w4849]
                                in-place-border: [w4846] -> w4838
                                n2023 = in-place-cluster #34(w4842) -> ("aAO"=w4848:u32[])
                                n2024 = call "remove channel from active arrayv2.vi"("line array in"=w4848, "line to remove"=w4849) -> ("line array out"=w4847:u32[], "index"=w4846:i32)  [unwired: 1 out]
                                n2025 = in-place-cluster #34("aAO"=w4847) -> (w4839:T12)
                                }
                                n2026 = call "2pparameters.vi"("Params in"=w4839, "command"="set") -> ()  [unwired: 1 out]
                                }
                                frame #1 {
                                n2027 = call "waveformparamsv2.vi"("command"="rem AO", "index"=w4850) -> ()  [unwired: 3 in, 3 out]
                                }
                                frame #2 {
                                n2028 = call "waveformsAObuffer.vi"("command"="get") -> ("AO wf out"=w4856:waveform(dbl)[])  [unwired: 1 in]
                                n2029 = Delete From Array(array=w4856, length=1, index=w4855) -> (array with subset deleted=w4852:waveform(dbl)[])  [unwired: 1 out]
                                n2030 = call "waveformsAObuffer.vi"("AO wf in"=w4852, "command"="set") -> ()  [unwired: 1 out]
                                }
                                }
                                }
                                frame False {
                                n2031 = stacked-sequence {
                                seq-local: [w4860 _ _] -> [_ w4868 w4879]
                                tunnel: w4859 -> [_ w4867 _]
                                tunnel: w4858 -> [_ _ w4878]
                                frame #0 {
                                n2032 = call "configuration.vi"("command"="get") -> ("config out"=w4865:T13)  [unwired: 2 in, 1 out]
                                n2033 = Unbundle By Name(w4865) -> ("Voltage to Ygalvo"=w4861:i32)
                                n2034 = call "2pparameters.vi"("command"="get") -> ("params out"=w4864:T12)  [unwired: 1 in]
                                n2035 = Unbundle By Name(w4864) -> ("aAO"=w4862:u32[])
                                n2036 = Search 1D Array(1D array=w4862, element=w4861) -> (index of element=w4860:i32)  [unwired: 1 in]
                                }
                                frame #1 {
                                n2037 = call "waveformparamsv2.vi"("command"="get") -> ("Params out"=w4871:T16)  [unwired: 4 in, 2 out]
                                n2038 = in-place {
                                in-place-border: w4868 -> [w4875]
                                in-place-border: w4867 -> [w4874]
                                n2039 = in-place-cluster #35(w4871) -> ("AO parameters"=w4876:T17)
                                n2040 = in-place {
                                in-place-border: w4874 -> [w4877]
                                n2041 = in-place-array #36(w4876, w4875) -> ()  [unwired: 1 out]
                                n2042 = in-place-array #36(w4877) -> (w4873:T17)  [unwired: 1 out]
                                }
                                n2043 = in-place-cluster #35("AO parameters"=w4873) -> (w4869:T16)
                                }
                                n2044 = call "waveformparamsv2.vi"("command"="set", "Params in"=w4869) -> ()  [unwired: 3 in, 3 out]
                                }
                                frame #2 {
                                n2045 = call "waveformsAObuffer.vi"("command"="get") -> ("AO wf out"=w4882:waveform(dbl)[])  [unwired: 1 in]
                                n2046 = Replace Array Subset(array=w4882, new element=w4878, index=w4879) -> (w4880:waveform(dbl)[])
                                n2047 = call "waveformsAObuffer.vi"("AO wf in"=w4880, "command"="set") -> ()  [unwired: 1 out]
                                }
                                }
                                }
                                }
                              }
                              frame #2 {
                                n2048 = Build Array(w4888, w4887) -> (w4889:bool[])
                                n2049 = Boolean Array To Number(Boolean array=w4889) -> (number=w4886:u32)
                                n2050 = case shown="2" w4886 {
                                tunnel: w4891 -> [_ _ w4934]
                                tunnel: w4890 -> [_ _ w4933]
                                tunnel: w4885 -> [_ w4913 w4932]
                                tunnel: w4884 -> [_ w4912 w4931]
                                frame 1, Default {
                                n2051 = stacked-sequence {
                                seq-local: [w4892 _ _] -> [_ w4904 w4909]
                                frame #0 {
                                n2052 = call "configuration.vi"("command"="get") -> ("config out"=w4898:T13)  [unwired: 2 in, 1 out]
                                n2053 = Unbundle By Name(w4898) -> ("2P shutter"=w4895:i32)
                                n2054 = call "2pparameters.vi"("command"="get") -> ("params out"=w4896:T12)  [unwired: 1 in]
                                n2055 = in-place {
                                in-place-border: w4895 -> [w4903]
                                in-place-border: [w4900] -> w4892
                                n2056 = in-place-cluster #37(w4896) -> ("aDO"=w4902:u32[])
                                n2057 = call "remove channel from active arrayv2.vi"("line array in"=w4902, "line to remove"=w4903) -> ("line array out"=w4901:u32[], "index"=w4900:i32)  [unwired: 1 out]
                                n2058 = in-place-cluster #37("aDO"=w4901) -> (w4893:T12)
                                }
                                n2059 = call "2pparameters.vi"("Params in"=w4893, "command"="set") -> ()  [unwired: 1 out]
                                }
                                frame #1 {
                                n2060 = call "waveformparamsv2.vi"("command"="rem DO", "index"=w4904) -> ()  [unwired: 3 in, 3 out]
                                }
                                frame #2 {
                                n2061 = call "waveformsDObuffer.vi"("command"="get") -> ("DO wf out"=w4910:digitalwaveform[])  [unwired: 1 in]
                                n2062 = Delete From Array(array=w4910, length=1, index=w4909) -> (array with subset deleted=w4906:digitalwaveform[])  [unwired: 1 out]
                                n2063 = call "waveformsDObuffer.vi"("DO wf in"=w4906, "command"="set") -> ()  [unwired: 1 out]
                                }
                                }
                                }
                                frame 2 {
                                n2064 = stacked-sequence {
                                tunnel: w4913 -> [_ w4924 _]
                                tunnel: w4912 -> [_ _ w4926]
                                frame #0 {
                                n2065 = call "configuration.vi"("command"="get") -> ("config out"=w4915:T13)  [unwired: 2 in, 1 out]
                                n2066 = call "2pparameters.vi"("command"="get") -> ("params out"=w4919:T12)  [unwired: 1 in]
                                n2067 = Unbundle By Name(w4915) -> ("2P shutter"=w4914:i32)
                                n2068 = in-place {
                                in-place-border: w4914 -> [w4923]
                                n2069 = in-place-cluster #38(w4919) -> ("aDO"=w4922:u32[])
                                n2070 = call "add channel to active arrayv2.vi"("line array in"=w4922, "line to add"=w4923) -> ("line array out"=w4921:u32[])  [unwired: 2 out]
                                n2071 = in-place-cluster #38("aDO"=w4921) -> (w4917:T12)
                                }
                                n2072 = call "2pparameters.vi"("Params in"=w4917, "command"="set") -> ()  [unwired: 1 out]
                                }
                                frame #1 {
                                n2073 = call "waveformparamsv2.vi"("command"="add DO", "add DO"=w4924) -> ()  [unwired: 3 in, 3 out]
                                }
                                frame #2 {
                                n2074 = call "waveformsDObuffer.vi"("command"="get") -> ("DO wf out"=w4929:digitalwaveform[])  [unwired: 1 in]
                                n2075 = Build Array (concatenate)(w4929, w4926) -> (w4928:digitalwaveform[])
                                n2076 = call "waveformsDObuffer.vi"("DO wf in"=w4928, "command"="set") -> ()  [unwired: 1 out]
                                }
                                }
                                }
                                frame 0 {
                                n2077 = stacked-sequence {
                                seq-local: [w4935 _ _] -> [_ w4943 w4965]
                                tunnel: w4934 -> [_ _ _]
                                tunnel: w4933 -> [_ _ _]
                                tunnel: w4932 -> [_ w4942 _]
                                tunnel: w4931 -> [_ _ w4964]
                                frame #0 {
                                n2078 = call "configuration.vi"("command"="get") -> ("config out"=w4940:T13)  [unwired: 2 in, 1 out]
                                n2079 = call "2pparameters.vi"("command"="get") -> ("params out"=w4939:T12)  [unwired: 1 in]
                                n2080 = Unbundle By Name(w4940) -> ("2P shutter"=w4936:i32)
                                n2081 = Unbundle By Name(w4939) -> ("aDO"=w4937:u32[])
                                n2082 = Search 1D Array(1D array=w4937, element=w4936) -> (index of element=w4935:i32)  [unwired: 1 in]
                                }
                                frame #1 {
                                n2083 = call "2pparameters.vi"("command"="get") -> ("params out"=w4946:T12)  [unwired: 1 in]
                                n2084 = Unbundle By Name(w4946) -> ("wavdet"=w4944:bool, "autoshutter"=w4945:bool)
                                n2085 = case shown="True" w4945 {
                                tunnel: w4943 -> [_ w4950]
                                tunnel: w4944 -> [_ w4949]
                                tunnel: w4942 -> [_ w4948]
                                frame False {
                                }
                                frame True {
                                n2086 = case shown="False" w4949 {
                                tunnel: w4950 -> [w4954 _]
                                tunnel: w4948 -> [w4951 _]
                                frame False {
                                n2087 = Index Array(array=w4951, index=0) -> (element=w4952:T20)
                                n2088 = call "waveformparamsv2.vi"("command"="get") -> ("Params out"=w4957:T16)  [unwired: 4 in, 2 out]
                                n2089 = in-place {
                                in-place-border: w4954 -> [w4961]
                                in-place-border: w4952 -> [w4959]
                                n2090 = in-place-cluster #39(w4957) -> ("DO parameters"=w4962:T19)
                                n2091 = in-place {
                                in-place-border: w4959 -> [w4963]
                                n2092 = in-place-array #40(w4962, w4961) -> ()  [unwired: 1 out]
                                n2093 = in-place-array #40(w4963) -> (w4960:T19)  [unwired: 1 out]
                                }
                                n2094 = in-place-cluster #39("DO parameters"=w4960) -> (w4955:T16)
                                }
                                n2095 = call "waveformparamsv2.vi"("command"="set", "Params in"=w4955) -> ()  [unwired: 3 in, 3 out]
                                }
                                frame True {
                                }
                                }
                                }
                                }
                                }
                                frame #2 {
                                n2096 = call "2pparameters.vi"("command"="get") -> ("params out"=w4968:T12)  [unwired: 1 in]
                                n2097 = Unbundle By Name(w4968) -> ("wavdet"=w4966:bool, "autoshutter"=w4967:bool)
                                n2098 = case shown="True" w4967 {
                                tunnel: w4965 -> [_ w4972]
                                tunnel: w4966 -> [_ w4971]
                                tunnel: w4964 -> [_ w4970]
                                frame False {
                                }
                                frame True {
                                n2099 = case shown="False" w4971 {
                                tunnel: w4972 -> [w4976 _]
                                tunnel: w4970 -> [w4974 _]
                                frame False {
                                n2100 = Index Array(array=w4974, index=0) -> (element=w4973:digitalwaveform)
                                n2101 = call "waveformsDObuffer.vi"("command"="get") -> ("DO wf out"=w4978:digitalwaveform[])  [unwired: 1 in]
                                n2102 = Replace Array Subset(array=w4978, new element=w4973, index=w4976) -> (w4980:digitalwaveform[])
                                n2103 = call "waveformsDObuffer.vi"("DO wf in"=w4980, "command"="set") -> ()  [unwired: 1 out]
                                }
                                frame True {
                                }
                                }
                                }
                                }
                                }
                                }
                                }
                                }
                              }
                              frame #3 {
                                n2104 = Build Array(w4983, w4982) -> (w4984:bool[])
                                n2105 = Boolean Array To Number(Boolean array=w4984) -> (number=w4981:u32)
                                n2106 = case shown="2" w4981 {
                                tunnel: w4988 -> [_ _ w5031]
                                tunnel: w4987 -> [_ _ w5030]
                                tunnel: w4986 -> [_ w5010 w5028]
                                tunnel: w4985 -> [_ w5009 w5029]
                                frame 1, Default {
                                n2107 = stacked-sequence {
                                seq-local: [w4989 _ _] -> [_ w5001 w5006]
                                frame #0 {
                                n2108 = call "configuration.vi"("command"="get") -> ("config out"=w4995:T13)  [unwired: 2 in, 1 out]
                                n2109 = Unbundle By Name(w4995) -> ("LT timestamp"=w4992:u32)
                                n2110 = call "2pparameters.vi"("command"="get") -> ("params out"=w4993:T12)  [unwired: 1 in]
                                n2111 = in-place {
                                in-place-border: w4992 -> [w5000]
                                in-place-border: [w4997] -> w4989
                                n2112 = in-place-cluster #41(w4993) -> ("aDO"=w4999:u32[])
                                n2113 = call "remove channel from active arrayv2.vi"("line array in"=w4999, "line to remove"=w5000) -> ("line array out"=w4998:u32[], "index"=w4997:i32)  [unwired: 1 out]
                                n2114 = in-place-cluster #41("aDO"=w4998) -> (w4990:T12)
                                }
                                n2115 = call "2pparameters.vi"("Params in"=w4990, "command"="set") -> ()  [unwired: 1 out]
                                }
                                frame #1 {
                                n2116 = call "waveformparamsv2.vi"("command"="rem DO", "index"=w5001) -> ()  [unwired: 3 in, 3 out]
                                }
                                frame #2 {
                                n2117 = call "waveformsDObuffer.vi"("command"="get") -> ("DO wf out"=w5007:digitalwaveform[])  [unwired: 1 in]
                                n2118 = Delete From Array(array=w5007, length=1, index=w5006) -> (array with subset deleted=w5003:digitalwaveform[])  [unwired: 1 out]
                                n2119 = call "waveformsDObuffer.vi"("DO wf in"=w5003, "command"="set") -> ()  [unwired: 1 out]
                                }
                                }
                                }
                                frame 2 {
                                n2120 = stacked-sequence {
                                tunnel: w5010 -> [_ _ w5023]
                                tunnel: w5009 -> [_ w5021 _]
                                frame #0 {
                                n2121 = call "configuration.vi"("command"="get") -> ("config out"=w5012:T13)  [unwired: 2 in, 1 out]
                                n2122 = Unbundle By Name(w5012) -> ("LT timestamp"=w5011:u32)
                                n2123 = call "2pparameters.vi"("command"="get") -> ("params out"=w5016:T12)  [unwired: 1 in]
                                n2124 = in-place {
                                in-place-border: w5011 -> [w5020]
                                n2125 = in-place-cluster #42(w5016) -> ("aDO"=w5019:u32[])
                                n2126 = call "add channel to active arrayv2.vi"("line array in"=w5019, "line to add"=w5020) -> ("line array out"=w5018:u32[])  [unwired: 2 out]
                                n2127 = in-place-cluster #42("aDO"=w5018) -> (w5014:T12)
